vi "statsCalcWriter.vi"(8 "error in (no error)":errorcluster, 10 "Output\nFilename":string, 11 "StatsCalc ID":i32) -> (0 "error out":errorcluster)   [LabVIEW 2014]
uses:
  <userlib>/StatsCalculatorLabView/StatsCalculatorLabView.lvlib
panel:
  out "Stripped \nVI Name":string
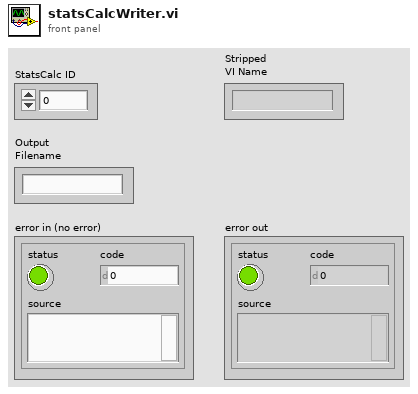
[diagram p1: front panel]
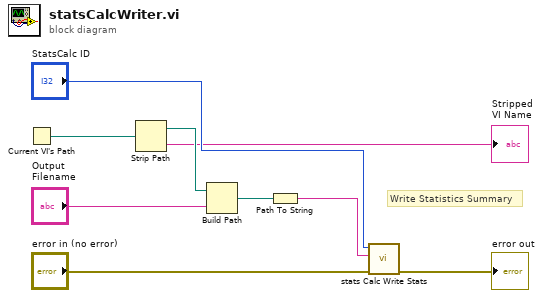
[diagram p0: block diagram]
diagram:
  # "Write Statistics Summary"
  n1 = Current VI's Path() -> (path=w1:path)
  n2 = Strip Path(path=w1) -> (stripped path=w3:path, name=→"Stripped \nVI Name":string)
  n3 = Build Path(base path=w3, name or relative path="Output\nFilename") -> (appended path=w5:path)
  n4 = Path To String(path=w5) -> (string=w6:string)
  n5 = call <userlib>:"stats Calc Write Stats.vi"("error in (no error)"="error in (no error)", "fileName"=w6, "handle"="StatsCalc ID") -> ("error out"=→"error out":errorcluster)  [unwired: 8 in]
